vi "kCoerceInt.vi"(8 "lower":i32, 9 "input":i32, 10 "upper":i32) -> (0 "coerced?":bool, 2 "output":i32)   [LabVIEW 2010, in "kevLib2011.lvlib"]
uses:
  kevLib2011.lvlib
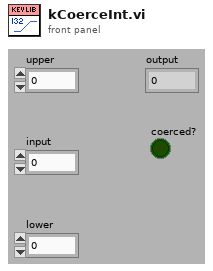
[diagram p1: front panel]
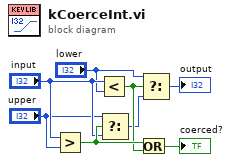
[diagram p0: block diagram]
diagram:
  n1 = Greater?(x="input", y="upper") -> (0:w7:bool)
  n2 = Less?(x="input", y="lower") -> (x < y?=w6:bool)
  n3 = Select(t="upper", s=w7, f="input") -> (s? t:f=w3:i32)
  n4 = Or(x=w7, y=w6) -> (x .or. y?=→"coerced?":bool)
  n5 = Select(t="lower", s=w6, f=w3) -> (s? t:f=→"output":i32)
